vi "Configure UDP Streaming.vi"(8 "error in (no error)":errorcluster, 9 "UDP Streaming Options":T1, 10 "UDP Streaming Port":u16=61557, 11 "PF_API in":refnum<class "PF_API.lvclass">) -> (0 "error out":errorcluster, 3 "PF_API out":refnum<class "PF_API.lvclass">)   [LabVIEW 2019, in "PF_API.lvclass"]
doc: "Configures the UPD communication on the selected port to get the data stream from the sensor. This VI also sets the angle start, maximum samples per scan and packet type."
uses:
  PF_API.lvclass
  Packet Classes/Packet A/Packet A.lvclass
  PF_API.lvclass/PF_API.ctl
  <vilib>/httpClient/POSTBuffer.vi
  <vilib>/httpClient/LabVIEWHTTPClient.lvlib
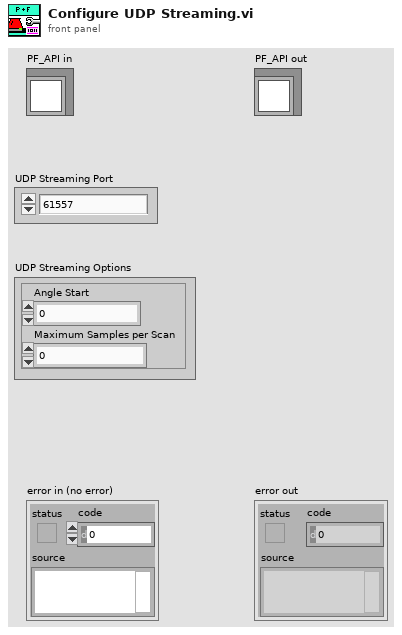
[diagram p1: front panel]
types:
  T1 = cluster{"Angle Start":i32, "Maximum Samples per Scan":u16}
  T2 = typedef "LabVIEWHTTPClient.lvlib/ClientHandle.ctl" = refnum<k1>
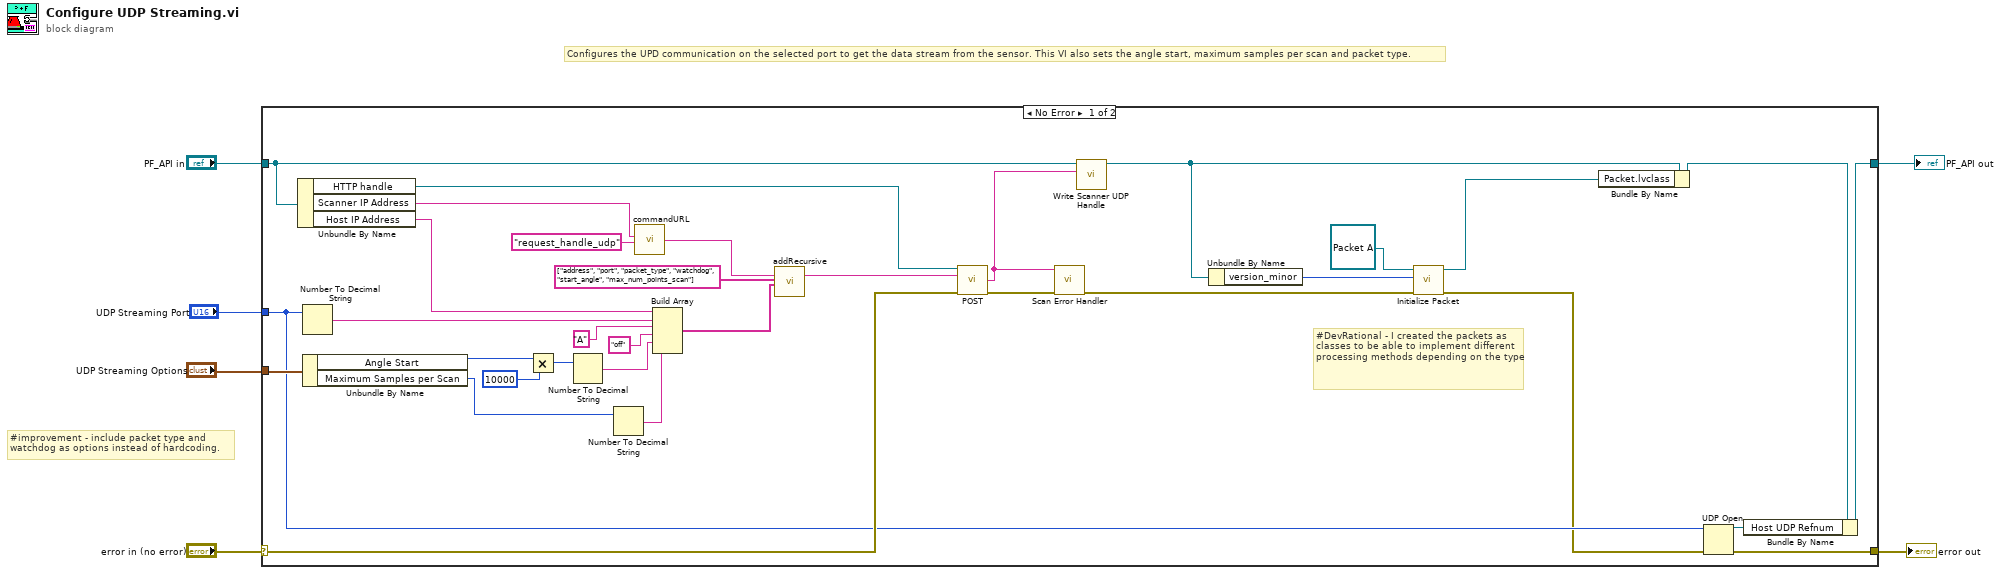
[diagram p0: block diagram]
diagram:
  # "#improvement - include packet type and\nwatchdog as options instead of hardcoding."
  # "Configures the UPD communication on the selected port to get the data stream from the sensor. This VI also sets the angle start, maximum samples per scan and packet type."
  n1 = case shown="No Error" "error in (no error)" {
    selector: "error in (no error)" -> [w39 w41]
    tunnel: [w19 w41] -> w5
    tunnel: [w17 w40] -> w3
    tunnel: "PF_API in" -> [w25 w40]
    tunnel: "UDP Streaming Options" -> [w36 _]
    tunnel: "UDP Streaming Port" -> [w18 _]
    frame No Error {
      # "#DevRational - I created the packets as classes to be able to implement different processing methods depending on the type"
      n2 = Unbundle By Name(w25) -> ("HTTP handle"=w22:T2, "Scanner IP Address"=w24:string, "Host IP Address"=w35:string)
      n3 = Number To Decimal String(number=w18) -> (decimal integer string=w34:string)  [unwired: 1 in]
      n4 = Unbundle By Name(w36) -> ("Angle Start"=w32:i32, "Maximum Samples per Scan"=w31:u16)
      n5 = Multiply(x=w32, y=10000 ("x")) -> (x*y=w8:i32)
      n6 = Number To Decimal String(number=w8) -> (decimal integer string=w30:string)  [unwired: 1 in]
      n7 = Number To Decimal String(number=w31) -> (decimal integer string=w29:string)  [unwired: 1 in]
      n8 = call "commandURL.vi"("Command String"="request_handle_udp" ("Scanner IP Address"), "Scanner IP Address"=w24) -> ("Command URL"=w38:string)  [unwired: 4 in]
      n9 = Build Array(w35, w34, "A" ("element"), "off" ("element"), w30, w29) -> (w28:string[])
      n10 = call "addRecursive.vi"("Command URL in"=w38, "Parameter Key"=string[] ["address", "port", "packet_type", "watchdog", "start_angle", "max_num_points_scan"], "Parameter Value"=w28) -> ("Command URL out"=w26:string)  [unwired: 13 in, 3 out]
      n11 = call-poly <vilib>:"POST.vi"("client handle"=w22, "url"=w26, "error in (no error)"=w39) -> ("body"=w20:string, "error out"=w27:errorcluster)  [unwired: 9 in, 2 out]
      n12 = call "Scan Error Handler.vi"("Error In"=w27, "HTTP Response"=w20) -> ("Error Out"=w21:errorcluster)  [unwired: 9 in]
      n13 = call "Write Scanner UDP Handle.vi"("HTTP response"=w20, "PF_API in"=w25) -> ("PF_API out"=w10:refnum<class "PF_API.lvclass">)  [unwired: 8 in, 1 out]
      n14 = Unbundle By Name(w10) -> ("version_minor"=w9:i32)
      n15 = call-dynamic "Initialize Packet.vi"("error in (no error)"=w21, "Protocol Version"=w9, "Packet A in"=refnum<class "Packet A.lvclass"> refnum ("Packet A.lvclass")) -> ("error out"=w14:errorcluster, "Packet A out"=w12:refnum<class "Packet A.lvclass">)  [unwired: 7 in]
      n16 = Bundle By Name(cluster=w10, "Packet.lvclass"=w12) -> (w15:refnum<class "PF_API.lvclass">)
      n17 = UDP Open(8:w14, 11:w18) -> (port=w16:refnum<k16>, 0:w19:errorcluster)  [unwired: 3 in, 1 out]
      n18 = Bundle By Name(cluster=w15, "Host UDP Refnum"=w16) -> (w17:refnum<class "PF_API.lvclass">)
    }
    frame Error {
    }
  }
  "error out" <- w5
  "PF_API out" <- w3
